vi "Check_data_ready.vi"(8 "Error_in":errorcluster, 11 "VISA in":refnum<visa-resource-name>) -> (0 "error out":errorcluster, 3 "VISA out":refnum<visa-resource-name>)   [LabVIEW 2019]
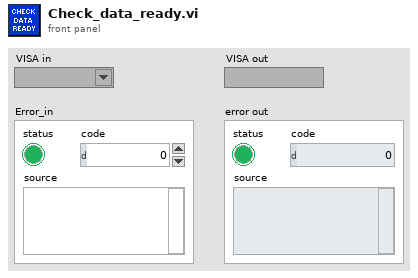
[diagram p1: front panel]
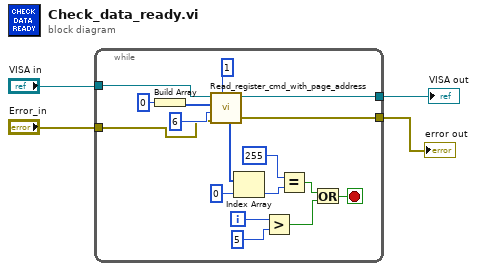
[diagram p0: block diagram]
diagram:
  n1 = while {
    tunnel: "VISA in" -> [w17]
    tunnel: "Error_in" -> [w16]
    tunnel: [w15] -> w3
    tunnel: [w14] -> w4
    i -> [w12]
    stop <- w9 stop-if-true
    n2 = Build Array(u8 0 ("element")) -> (w21:u8[])
    n3 = call "Read_register_cmd_with_page_address.vi"("Words_to_read"=u16 1, "error in (no error)"=w16, "Register Address"=u8 6, "Page address"=w21, "VISA Refnum in"=w17) -> ("error out"=w14:errorcluster, "VISA Refnum out"=w15:refnum<visa-resource-name>, "RdReg Data"=w8:u8[])  [unwired: 4 in]
    n4 = Index Array(array=w8, index=0) -> (element=w6:u8)
    n5 = Greater?(x=w12, y=5) -> (0:w10:bool)
    n6 = Equal?(x=u8 255, y=w6) -> (x = y?=w13:bool)
    n7 = Or(x=w13, y=w10) -> (x .or. y?=w9:bool)
  }
  "error out" <- w4
  "VISA out" <- w3
